vi "Get_Comaptibility_Mode.vi"(8 "error in (no error)":errorcluster, 11 "AB_InteropAssembly in":refnum<class "AB_InteropAssembly.lvclass">) -> (0 "error out":errorcluster, 2 "CompatibilityWith2011":bool, 3 "AB_InteropAssembly out":refnum<class "AB_InteropAssembly.lvclass">)   [LabVIEW 2020, in "AB_InteropAssembly.lvclass"]
uses:
  <vilib>/AppBuilder/AB_Classes/InteropAssembly/AB_InteropAssembly.lvclass
  <vilib>/AppBuilder/AB_Classes/InteropAssembly/AB_InteropAssembly.lvclass/AB_InteropAssembly.ctl
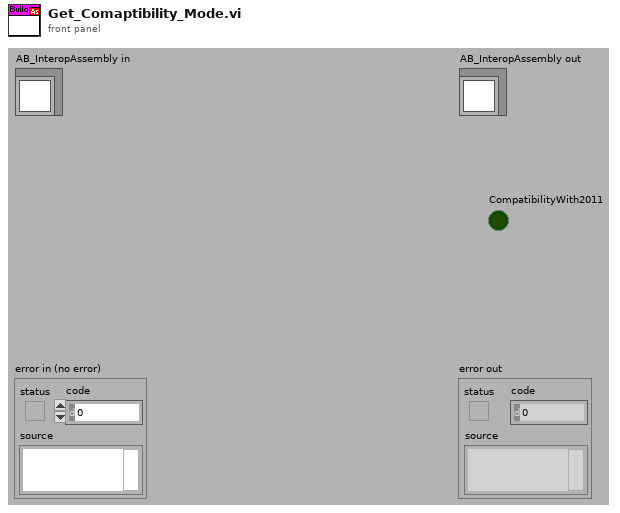
[diagram p1: front panel]
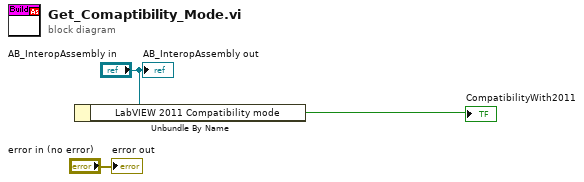
[diagram p0: block diagram]
diagram:
  n1 = Unbundle By Name("AB_InteropAssembly in") -> ("LabVIEW 2011 Compatibility mode"=→"CompatibilityWith2011":bool)
  "error out" <- "error in (no error)"
  "AB_InteropAssembly out" <- "AB_InteropAssembly in"
